vi "PowerSlideDrive.vi"(8 "error in (no error)":errorcluster, 11 "RobotDriveDevRef 2":T1={"DevStatus"={"status"=FALSE, "code"=0, "source"=""}, "Motors[]"=[], "Square Inputs"=FALSE, "Max Output"=1.0}) -> (0 "error out":errorcluster, 2 "Motor Values":dbl[](array[numeric]), 3 "RobotDriveDevRef":T1={"DevStatus"={"status"=FALSE, "code"=0, "source"=""}, "Motors[]"=[], "Square Inputs"=FALSE, "Max Output"=1.0})   [LabVIEW 2014, in "PowerSlide.lvlib"]
uses:
  PowerSlide.lvlib
  <vilib>/Rock Robotics/WPI/RobotDrive/WPI_RobotDriveDevRef.ctl
  <vilib>/Rock Robotics/WPI/MotorControl/WPI_MotorControlDeviceRef.ctl
  <vilib>/Rock Robotics/WPI/MotorControl/WPI_MotorControlType.ctl
  <vilib>/Rock Robotics/SystemInterfaces/Typedef/FPGA_TypedefDigitalModule.ctl
  <vilib>/Rock Robotics/SystemInterfaces/DIO/FPGA_DIOPWMChannel.ctl
  <vilib>/Rock Robotics/WPI/PWM/WPI_PWMDeadband.ctl
  <vilib>/Rock Robotics/WPI/CAN/Jaguar/SubVIs/WPI_CANJaguar_ControlMode.ctl
  <vilib>/Rock Robotics/WPI/CAN/TalonSRX/WPI_CANTalonSRX_APIControlMode.ctl
  <vilib>/Rock Robotics/WPI/PWM/WPI_PWMTransform_ConPane.ctl
panel:
  in  "RightSpeed":dbl
  in  "LeftSpeed":dbl
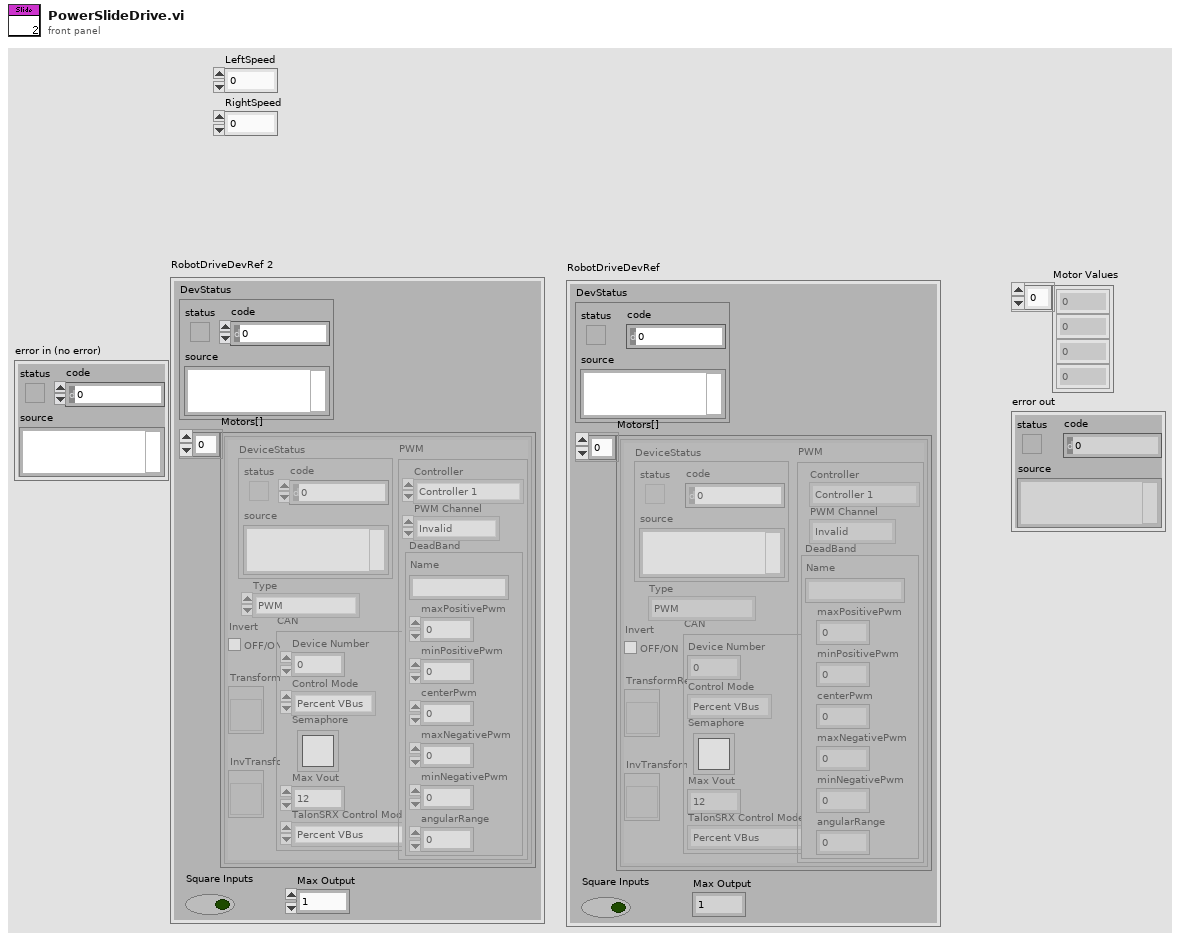
[diagram p1: front panel]
types:
  T1 = typedef "WPI_RobotDriveDevRef.ctl" = cluster{"DevStatus":errorcluster, "Motors[]":T2[], "Square Inputs":bool, "Max Output":dbl}
  T2 = typedef "WPI_MotorControlDeviceRef.ctl" = cluster{"DeviceStatus":errorcluster, "Type":T3, "PWM":cluster{"Controller":T4, "PWM Channel":T5, "DeadBand":T6}, "CAN":cluster{"Device Number":u8, "Control Mode":T7, "Semaphore":T8, "Max Vout":dbl, "TalonSRX Control Mode":T9}, "Invert":bool, "TransformRef":T10, "InvTransformRef":T10}
  T3 = typedef "WPI_MotorControlType.ctl" = enum16{"PWM", "CAN", "CANTalonSRX"}
  T4 = typedef "FPGA_TypedefDigitalModule.ctl" = enum16{"Controller 1"}
  T5 = typedef "FPGA_DIOPWMChannel.ctl" = enum8{"PWM 0", "PWM 1", "PWM 2", "PWM 3", "PWM 4", "PWM 5", "PWM 6", "PWM 7", "PWM 8", "PWM 9", "PWM MXP 0", "PWM MXP 1", "PWM MXP 2", "PWM MXP 3", "PWM MXP 4", "PWM MXP 5", "PWM MXP 6", "PWM MXP 7", "PWM MXP 8", "PWM MXP 9", "Invalid"}
  T6 = typedef "WPI_PWMDeadband.ctl" = cluster{"Name":string, "maxPositivePwm":i32, "minPositivePwm":i32, "centerPwm":i32, "maxNegativePwm":i32, "minNegativePwm":i32, "angularRange":u16}
  T7 = typedef "WPI_CANJaguar_ControlMode.ctl" = enum8{"Percent VBus", "Current", "Speed", "Position", "Voltage"}
  T8 = typedef "Semaphore RefNum" = refnum<k1>
  T9 = typedef "WPI_CANTalonSRX_APIControlMode.ctl" = enum8{"Percent VBus", "Speed", "Position", "Slave", "Unchanged / Invalid"}
  T10 = typedef "WPI_PWMTransform_ConPane.ctl" = refnum<vi>
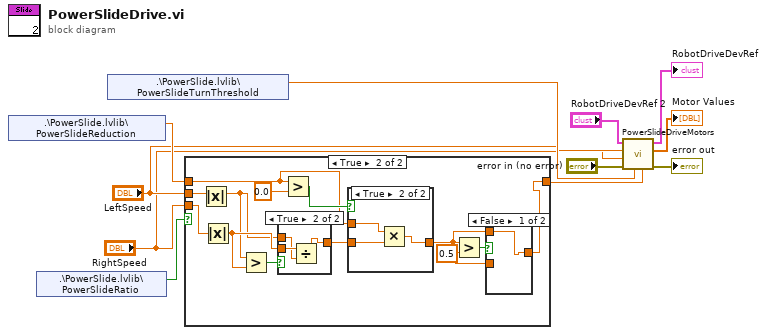
[diagram p0: block diagram]
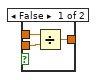
[diagram p5: hidden frame]
diagram:
  n1 = shared-variable ".\\PowerSlide.lvlib\\PowerSlideReduction"() -> (w4:dbl)  [unwired: 1 in, 1 out]
  n2 = shared-variable ".\\PowerSlide.lvlib\\PowerSlideRatio"() -> (w6:bool)  [unwired: 1 in, 1 out]
  n3 = shared-variable ".\\PowerSlide.lvlib\\PowerSlideTurnThreshold"() -> (w3:dbl)  [unwired: 1 in, 1 out]
  n4 = case shown="True" w6 {
    tunnel: [w12 w13] -> w5
    tunnel: w4 -> [w12 w21]
    tunnel: "LeftSpeed" -> [_ w18]
    tunnel: "RightSpeed" -> [_ w20]
    frame False {
    }
    frame True {
      w15 = 0.5 ("y")
      n5 = Absolute Value(x=w18) -> (abs(x)=w17:dbl)
      n6 = Absolute Value(x=w20) -> (abs(x)=w19:dbl)
      n7 = Greater?(x=w17, y=w19) -> (0:w25:bool)
      n8 = case shown="True" w25 {
        tunnel: w19 -> [w34 w37]
        tunnel: w17 -> [w33 w36]
        tunnel: [w32 w35] -> w22
        frame False {
          n9 = Divide(x=w33, y=w34) -> (x/y=w32:dbl)
        }
        frame True {
          n10 = Divide(x=w37, y=w36) -> (x/y=w35:dbl)
        }
      }
      n11 = Greater?(x=w21, y=0.0) -> (0:w23:bool)
      n12 = case shown="True" w23 {
        tunnel: w22 -> [w28 w31]
        tunnel: w21 -> [_ w30]
        tunnel: [w28 w29] -> w14
        frame False {
        }
        frame True {
          n13 = Multiply(x=w30, y=w31) -> (x*y=w29:dbl)
        }
      }
      n14 = Greater?(x=w14, y=w15) -> (0:w16:bool)
      n15 = case shown="False" w16 {
        tunnel: [w26 w27] -> w13
        tunnel: w15 -> [_ w27]
        tunnel: w14 -> [w26 _]
        frame False {
        }
        frame True {
        }
      }
    }
  }
  n16 = call "PowerSlideDriveMotors.vi"("Reduction"=w5, "TurnThreshold"=w3, "error in (no error)"="error in (no error)", "RightSpeed"="RightSpeed", "LeftSpeed"="LeftSpeed", "RobotDriveDevRef 2"="RobotDriveDevRef 2") -> ("error out"=→"error out":errorcluster, "Motor Values"=→"Motor Values":dbl[], "RobotDriveDevRef"=→"RobotDriveDevRef":T1)  [unwired: 3 in]
